vi "vi.BufferReaderTemplate.vi"(8 "error in (no error)":errorcluster, 11 "BufferIn":string) -> (0 "error out":errorcluster)   [LabVIEW 2014, in "GLue.lvlib" / "class.GLue.lvclass"]
uses:
  class.GLue.lvclass
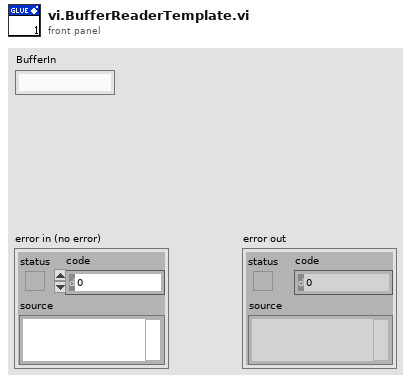
[diagram p1: front panel]
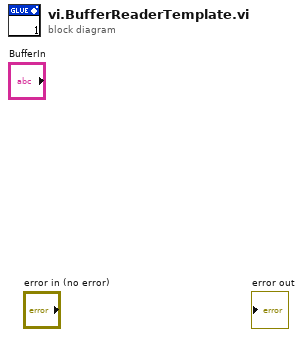
[diagram p0: block diagram]
diagram:
